vi "Draw Border.vi"(8 "error in (no error)":errorcluster, 11 "Triangle in":refnum<class "Triangle.lvclass">) -> (0 "error out":errorcluster, 2 "Picture out":picture, 3 "Triangle out":refnum<class "Triangle.lvclass">)   [LabVIEW 2015, in "Triangle.lvclass"]
uses:
  Triangle.lvclass
  Rectangle Border/Rectangle Border.lvclass
  Graphic/Graphic.lvclass/Graphic.ctl
  Rectangle Border/Rectangle Border.lvclass/Rectangle Border.ctl
  Scalable Border/Scalable Border.lvclass
  Graphic/Graphic.lvclass
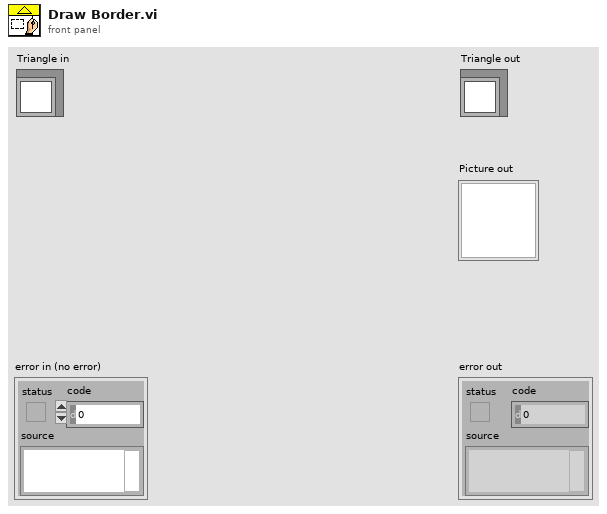
[diagram p1: front panel]
types:
  T1 = cluster{"Width":i16, "Style":enum32{"Solid", "Dash", "Dot", "DashDot", "DashDotDot"}}
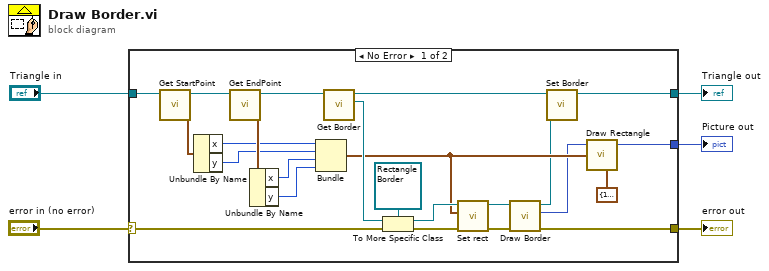
[diagram p0: block diagram]
diagram:
  n1 = case shown="No Error" "error in (no error)" {
    selector: "error in (no error)" -> [w15 w31]
    tunnel: [w14 w31] -> w3
    tunnel: [w9 _] -> w2
    tunnel: "Triangle in" -> [w13 w30]
    tunnel: [w7 w30] -> w1
    frame No Error {
      n2 = call "Get StartPoint.vi"("Graphic in"=w13) -> ("StartPoint"=w22:cluster{"x":i16, "y":i16}, "Graphic out"=w24:refnum<class "Triangle.lvclass">)  [unwired: 8 in, 1 out]
      n3 = Unbundle By Name(w22) -> ("x"=w20:i16, "y"=w19:i16)
      n4 = call "Get EndPoint.vi"("Graphic in"=w24) -> ("EndPoint"=w21:cluster{"x":i16, "y":i16}, "Graphic out"=w23:refnum<class "Triangle.lvclass">)  [unwired: 8 in, 1 out]
      n5 = Unbundle By Name(w21) -> ("x"=w18:i16, "y"=w17:i16)
      n6 = Bundle("x"=w20, "y"=w19, "x"=w18, "y"=w17) -> (w11:cluster{"x":i16, "y":i16, "x":i16, "y":i16})  [unwired: 1 in]
      n7 = call "Get Border.vi"("Graphic in"=w23) -> ("Scalable Border.lvclass"=w28:refnum<class "Scalable Border.lvclass">, "Graphic out"=w12:refnum<class "Triangle.lvclass">)  [unwired: 8 in, 1 out]
      n8 = To More Specific Class(target class=refnum<class "Rectangle Border.lvclass"> refnum ("Rectangle Border.lvclass"), reference=w28, error in=w15) -> (specific class reference=w26:refnum<class "Rectangle Border.lvclass">, error out=w27:errorcluster)
      n9 = call "Set rect.vi"("error in (no error)"=w27, "rect"=w11, "Rectangle Border in"=w26) -> ("error out"=w16:errorcluster, "Rectangle Border out"=w29:refnum<class "Rectangle Border.lvclass">)  [unwired: 7 in]
      n10 = call-dynamic "Draw Border.vi"("error in (no error)"=w16, "Rectangle Border in"=w29) -> ("error out"=w14:errorcluster, "Border out"=w10:picture, "Rectangle Border out"=w6:refnum<class "Rectangle Border.lvclass">)  [unwired: 7 in]
      n11 = call "Set Border.vi"("Scalable Border.lvclass"=w6, "Graphic in"=w12) -> ("Graphic out"=w7:refnum<class "Triangle.lvclass">)  [unwired: 8 in, 1 out]
      n12 = call <vilib>:"Draw Rectangle.vi"("picture"=w10, "rect"=w11, "pen"=T1 {"Width"=1, "Style"=enum."Dot"}) -> ("new picture"=w9:picture)  [unwired: 6 in]
    }
    frame Error {
    }
  }
  "error out" <- w3
  "Triangle out" <- w1
  "Picture out" <- w2
